vi "Gamma jj'.vi"(4 "X/Y":bool, 5 "error in (no error)":errorcluster, 6 "j' (1)":i32=1, 7 "j (1)":i32=1) -> (0 "error out":errorcluster, 1 "m'":i32, 2 "m":i32, 3 "Gamma Magnitude":dbl)   [LabVIEW 2020, in "Zernike Polynome.lvlib"]
doc: "This VI calculates the Zernike polynomial derivative matrix elements."
uses:
  Zernike Polynome.lvlib
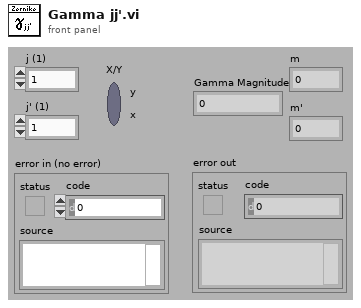
[diagram p1: front panel]
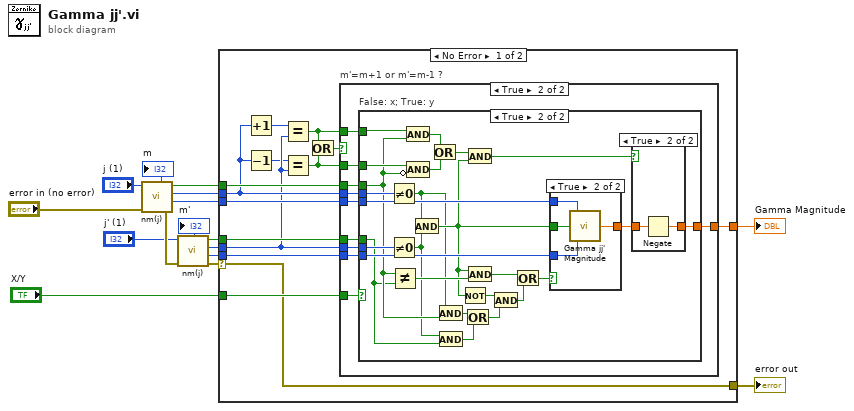
[diagram p0: block diagram]
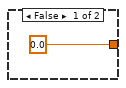
[diagram p2: hidden frame]
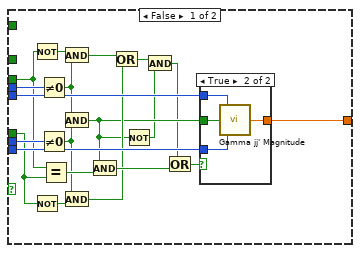
[diagram p3: hidden frame]
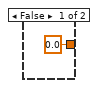
[diagram p4: hidden frame]
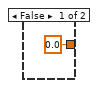
[diagram p6: hidden frame]
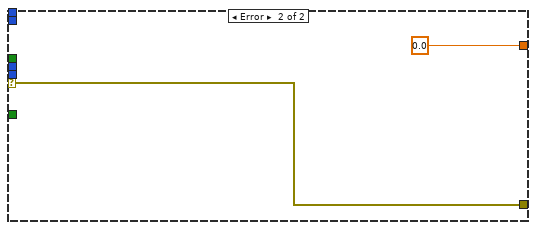
[diagram p7: hidden frame]
diagram:
  n1 = call "nm(j).vi"("error in (no error)"="error in (no error)", "j (1)"="j (1)") -> ("error out"=w14:errorcluster, "n"=w11:i32, "m"=w6:i32, "odd"=w8:bool)  [unwired: 2 in]
  "m" <- w6
  n2 = call "nm(j).vi"("error in (no error)"=w14, "j (1)"="j' (1)") -> ("error out"=w2:errorcluster, "n"=w10:i32, "m"=w5:i32, "odd"=w7:bool)  [unwired: 2 in]
  "m'" <- w5
  n3 = case shown="No Error" w2 {
    selector: w2 -> [w15 w99]
    tunnel: [w28 0.0 ("Magnitude")] -> w12
    tunnel: w11 -> [w27 _]
    tunnel: w10 -> [w26 _]
    tunnel: w8 -> [w25 _]
    tunnel: w7 -> [w24 _]
    tunnel: w6 -> [w23 _]
    tunnel: w5 -> [w22 _]
    tunnel: "X/Y" -> [w20 _]
    tunnel: [w15 w99] -> w1
    frame No Error {
      n4 = Increment(x=w23) -> (x+1=w19:i32)
      n5 = Decrement(x=w23) -> (x-1=w18:i32)
      n6 = Equal?(x=w19, y=w22) -> (x = y?=w16:bool)
      n7 = Equal?(x=w18, y=w22) -> (x = y?=w17:bool)
      n8 = Or(x=w16, y=w17) -> (x .or. y?=w21:bool)
      n9 = case "m'=m+1 or m'=m-1 ?" shown="True" w21 {
        tunnel: [0.0 ("Magnitude") w39] -> w28
        tunnel: w27 -> [_ w38]
        tunnel: w26 -> [_ w37]
        tunnel: w23 -> [_ w36]
        tunnel: w22 -> [_ w35]
        tunnel: w25 -> [_ w34]
        tunnel: w24 -> [_ w33]
        tunnel: w20 -> [_ w32]
        tunnel: w17 -> [_ w31]
        tunnel: w16 -> [_ w30]
        frame False {
        }
        frame True {
          n10 = case "False: x; True: y" shown="True" w32 {
            tunnel: [w59 w81] -> w39
            tunnel: w38 -> [w58 w89]
            tunnel: w37 -> [w57 w88]
            tunnel: w36 -> [w56 w87]
            tunnel: w35 -> [w55 w86]
            tunnel: w34 -> [w52 w69]
            tunnel: w33 -> [w47 w65]
            tunnel: w31 -> [_ w76]
            tunnel: w30 -> [_ w78]
            frame False {
              n11 = Not(x=w52) -> (.not. x?=w51:bool)
              n12 = Not(x=w47) -> (.not. x?=w48:bool)
              n13 = Not Equal To 0?(x=w56) -> (x != 0?=w50:bool)
              n14 = Not Equal To 0?(x=w55) -> (x != 0?=w46:bool)
              n15 = Equal?(x=w52, y=w47) -> (x = y?=w49:bool)
              n16 = And(x=w51, y=w50) -> (x .and. y?=w45:bool)
              n17 = And(x=w50, y=w46) -> (x .and. y?=w42:bool)
              n18 = And(x=w46, y=w48) -> (x .and. y?=w44:bool)
              n19 = And(x=w42, y=w49) -> (x .and. y?=w53:bool)
              n20 = Or(x=w45, y=w44) -> (x .or. y?=w43:bool)
              n21 = Not(x=w42) -> (.not. x?=w41:bool)
              n22 = And(x=w43, y=w41) -> (x .and. y?=w40:bool)
              n23 = Or(x=w40, y=w53) -> (x .or. y?=w54:bool)
              n24 = case shown="True" w54 {
                tunnel: [0.0 ("Magnitude") w64] -> w59
                tunnel: w58 -> [_ w63]
                tunnel: w57 -> [_ w62]
                tunnel: w42 -> [_ w61]
                frame False {
                }
                frame True {
                  n25 = call "Gamma jj' Magnitude.vi"("n'"=w62, "m,m' != 0"=w61, "n"=w63) -> ("Magnitude"=w64:dbl)
                }
              }
            }
            frame True {
              n26 = Not Equal To 0?(x=w87) -> (x != 0?=w68:bool)
              n27 = Not Equal To 0?(x=w86) -> (x != 0?=w66:bool)
              n28 = Not Equal?(x=w69, y=w65) -> (x != y?=w82:bool)
              n29 = And(x=w78, y=w69) -> (x .and. y?=w77:bool)
              n30 = Compound Arithmetic op=AND(w76, invert w69) -> (w75:bool)
              n31 = And(x=w68, y=w66) -> (x .and. y?=w73:bool)
              n32 = Or(x=w77, y=w75) -> (x .or. y?=w74:bool)
              n33 = And(x=w68, y=w69) -> (x .and. y?=w71:bool)
              n34 = And(x=w66, y=w65) -> (x .and. y?=w67:bool)
              n35 = Not(x=w73) -> (.not. x?=w79:bool)
              n36 = Or(x=w71, y=w67) -> (x .or. y?=w70:bool)
              n37 = And(x=w74, y=w73) -> (x .and. y?=w72:bool)
              n38 = And(x=w73, y=w82) -> (x .and. y?=w84:bool)
              n39 = And(x=w79, y=w70) -> (x .and. y?=w85:bool)
              n40 = Or(x=w84, y=w85) -> (x .or. y?=w83:bool)
              n41 = case shown="True" w83 {
                tunnel: [0.0 ("Magnitude") w97] -> w80
                tunnel: w89 -> [_ w96]
                tunnel: w88 -> [_ w95]
                tunnel: w73 -> [_ w94]
                frame False {
                }
                frame True {
                  n42 = call "Gamma jj' Magnitude.vi"("n'"=w95, "m,m' != 0"=w94, "n"=w96) -> ("Magnitude"=w97:dbl)
                }
              }
              n43 = case shown="True" w72 {
                tunnel: [w90 w92] -> w81
                tunnel: w80 -> [w90 w91]
                frame False {
                }
                frame True {
                  n44 = Negate(x=w91) -> (-x=w92:dbl)
                }
              }
            }
          }
        }
      }
    }
    frame Error {
    }
  }
  "error out" <- w1
  "Gamma Magnitude" <- w12
